vi "Write Configuration Parameter.vi"(8 "error in (no error)":errorcluster, 10 "Configuration":T1, 11 "RandomNumberGenerator in":refnum<class "RandomNumberGenerator.lvclass">) -> (0 "error out":errorcluster, 3 "RandomNumberGenerator out":refnum<class "RandomNumberGenerator.lvclass">)   [LabVIEW 2020, in "RandomNumberGenerator.lvlib" / "RandomNumberGenerator.lvclass"]
uses:
  RandomNumberGenerator.lvclass
  RandomNumberGenerator.lvclass/RandomNumberGenerator.ctl
  Configuration.ctl
panel:
  # "#via_ignore"
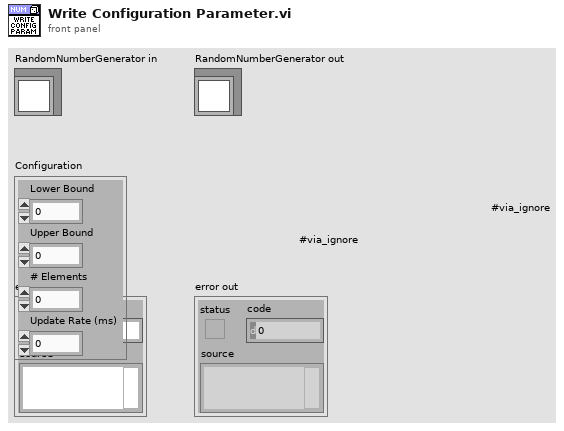
[diagram p1: front panel]
types:
  T1 = typedef "RandomNumberGenerator.lvlib/RandomNumberGenerator.lvclass/Configuration.ctl" = cluster{"Lower Bound":dbl, "Upper Bound":dbl, "# Elements":i32, "Update Rate (ms)":i32}
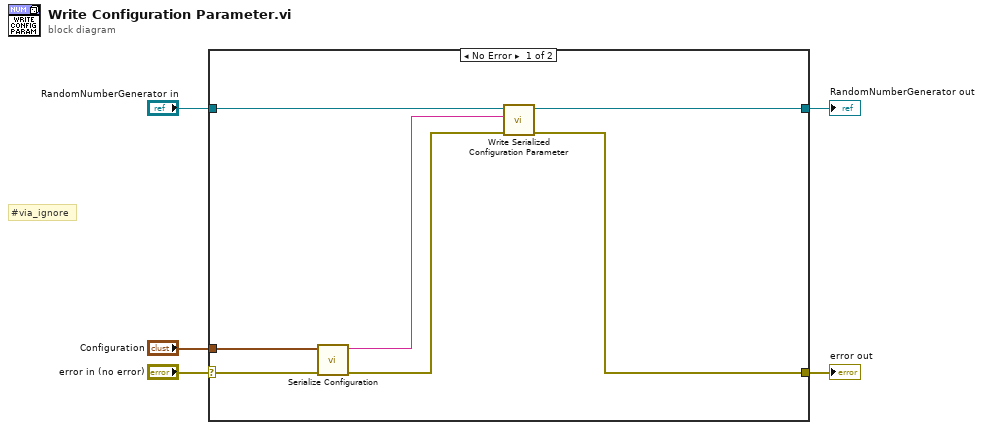
[diagram p0: block diagram]
diagram:
  # "#via_ignore"
  n1 = case shown="No Error" "error in (no error)" {
    selector: "error in (no error)" -> [w10 w14]
    tunnel: [w7 w14] -> w4
    tunnel: [w11 w13] -> w2
    tunnel: "RandomNumberGenerator in" -> [w12 w13]
    tunnel: "Configuration" -> [w6 _]
    frame No Error {
      n2 = call "Serialize Configuration.vi"("error in (no error)"=w10, "Configuration"=w6) -> ("error out"=w8:errorcluster, "Serialized Configuration"=w9:string)  [unwired: 8 in]
      n3 = call "Write Serialized Configuration Parameter.vi"("error in (no error)"=w8, "Serialized Configuration"=w9, "RandomNumberGenerator in"=w12) -> ("error out"=w7:errorcluster, "RandomNumberGenerator out"=w11:refnum<class "RandomNumberGenerator.lvclass">)  [unwired: 7 in]
    }
    frame Error {
    }
  }
  "error out" <- w4
  "RandomNumberGenerator out" <- w2
